vi "SampleAccumulator.vi"(7 "Write Element Data":T4={"Write Index"=0, "Write Element"=0, "Write?"=TRUE}, 8 "Input Valid":bool=TRUE, 9 "Acquisition Status In":T1, 11 "Input Data":T2=[0, 0, 0, 0]) -> (0 "End of Acc?":bool, 1 "Line Status Out":T3, 2 "Final Count":i16, 3 "Accumulated Value":i32[](array[numeric]), 5 "IsCurrentMaskNeg?":bool)   [LabVIEW 2014]
uses:
  <vilib>/rvi/FXPMathLib/basic elements/FxpDiscreteDelay/XNode/nifxpmath_DiscreteDelay.xnode
  <vilib>/rvi/DataTransferAndStorage/Container/XNode/niFpgaContainer.xnode
  <vilib>/rvi/interface/RandomDataEmulation/nirviRandomDataFpgaReadWriteTemplate.vi
  Adapter Module Specific/Multi-Channel Analog Input Data.ctl
  Acquisition Engine/Acquisition Status.ctl
panel:
  # "Copyright 2014 Vidrio Technologies\nScanImage 5 software is licensed under the Apache License, Version 2.0 (the \"License\"); you may not use any files contained\nwithin the ScanImage 5 release except in compliance with the License. You may obtain a copy of the License at\n http://www.apache.org/licenses/LICENSE-2.0\nUnless required by applicable law or agreed to in writing, software distributed under the License is distributed on an\n\"AS IS\" BASIS, WITHOUT WARRANTIES OR CONDITIONS OF ANY KIND, either express or implied. See the License for the\n specific language governing permissions and limitations under the License."
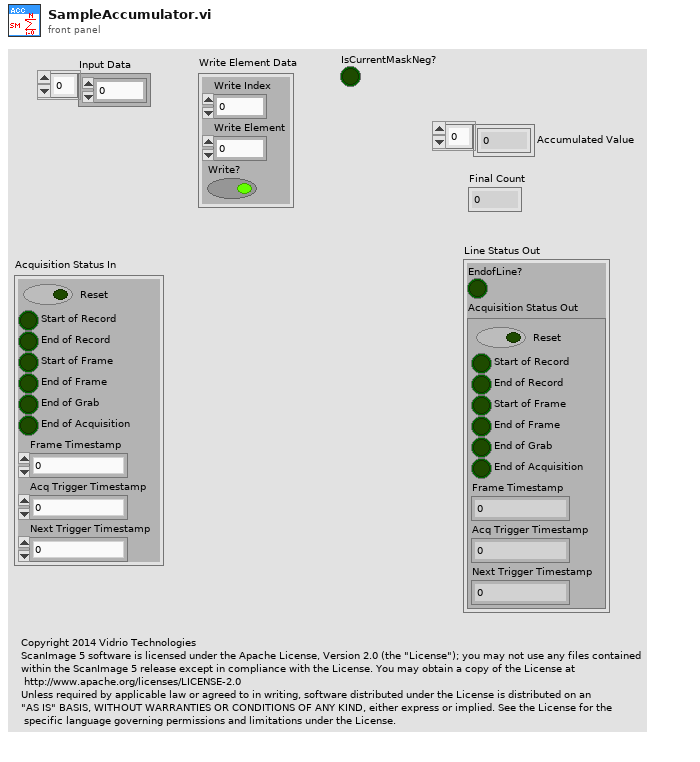
[diagram p1: front panel]
types:
  T1 = typedef "Acquisition Status.ctl" = cluster{"Reset":bool, "Start of Record":bool, "End of Record":bool, "Start of Frame":bool, "End of Frame":bool, "End of Grab":bool, "End of Acquisition":bool, "Frame Timestamp":u64, "Acq Trigger Timestamp":u64, "Next Trigger Timestamp":u64}
  T2 = typedef "Multi-Channel Analog Input Data.ctl" = i16[]
  T3 = cluster{"EndofLine?":bool, "Acquisition Status Out":T1}
  T4 = cluster{"Write Index":i32, "Write Element":i16, "Write?":bool}
  T5 = cluster{"Reset":bool, "Start of Record":bool, "End of Record":bool, "Start of Frame":bool, "End of Frame":bool, "End of Grab":bool, "End of Acquisition":bool, "Frame Timestamp":u64, "Acq Trigger Timestamp":u64, "Next Trigger Timestamp":u64}
  T6 = cluster{bool, "Q":cluster{"Reset":bool, "Start of Record":bool, "End of Record":bool, "Start of Frame":bool, "End of Frame":bool, "End of Grab":bool, "End of Acquisition":bool, "Frame Timestamp":u64, "Acq Trigger Timestamp":u64, "Next Trigger Timestamp":u64}}
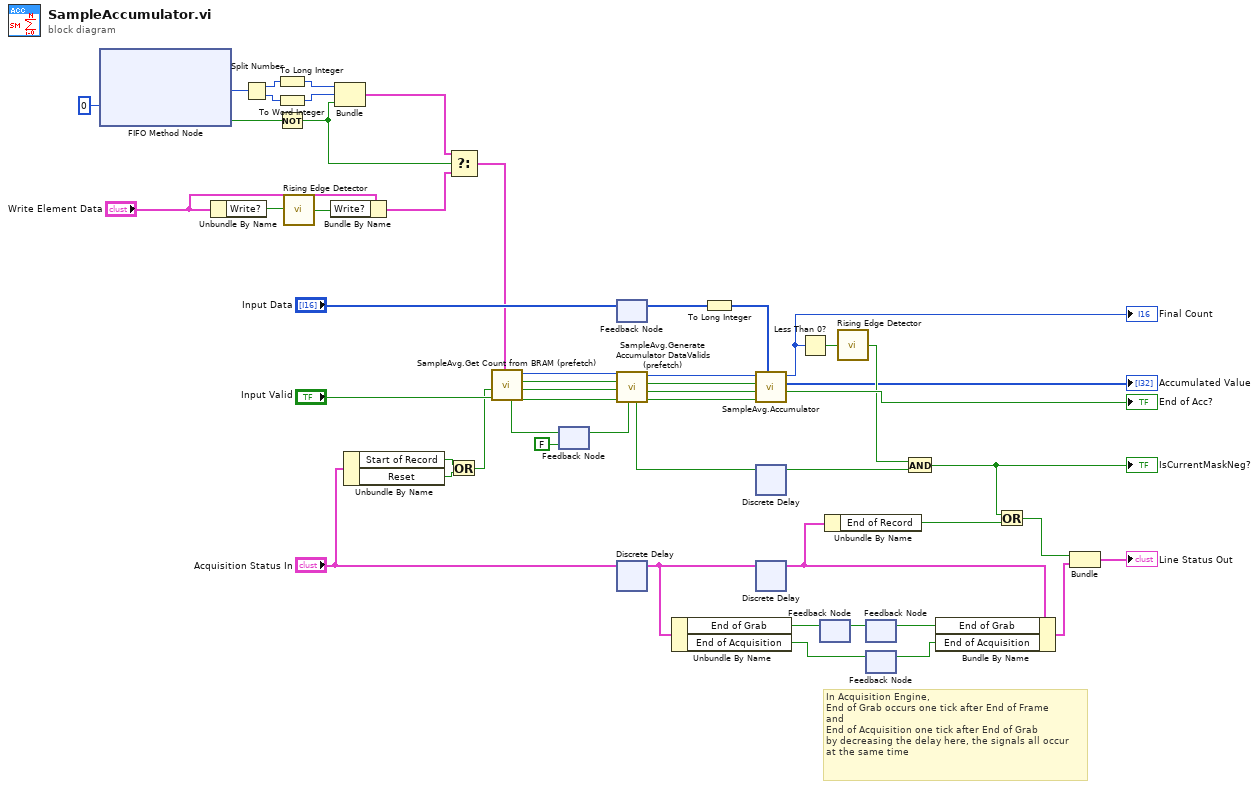
[diagram p0: block diagram]
diagram:
  # "In Acquisition Engine,\nEnd of Grab occurs one tick after End of Frame\nand\nEnd of Acquisition one tick after End of Grab\nby decreasing the delay here, the signals all occur\nat the same time"
  n1 = xnode ("FIFO Method Node")("Timeout"=0) -> ("Element"=w26:u32, "Timed Out?"=w23:bool)  [unwired: 1 in, 1 out]
  n2 = Unbundle By Name("Write Element Data") -> ("Write?"=w20:bool)
  n3 = Split Number(x=w26) -> (hi(x)=w22:u16, lo(x)=w25:u16)
  n4 = To Long Integer(number=w22) -> (32bit integer=w21:i32)
  n5 = To Word Integer(number=w25) -> (16bit integer=w24:i16)
  n6 = Not(x=w23) -> (.not. x?=w15:bool)
  n7 = call "Rising Edge Detector.vi"("signal"=w20) -> ("edge detected"=w18:bool)  [unwired: 14 in]
  n8 = Bundle By Name(cluster="Write Element Data", "Write?"=w18) -> (w17:T4)
  n9 = Bundle(w21, w24, w15) -> (w16:cluster{i32, i16, bool})  [unwired: 1 in]
  n10 = Unbundle By Name("Acquisition Status In") -> ("Start of Record"=w2:bool, "Reset"=w3:bool)
  n11 = Select(t=w16, s=w15, f=w17) -> (s? t:f=w14:T4)
  n12 = Or(x=w2, y=w3) -> (x .or. y?=w1:bool)
  n13 = feedback #1(FALSE ("Get New Load")) -> (w50:bool)
  n14 = call "SampleAvg.Get Count from BRAM (prefetch).vi"("Step?"=w50, "Write Element Data"=w14, "Input Valid"="Input Valid", "Start New Record"=w1) -> ("Output Valid"=w52:bool, "Start of New Record"=w47:bool, "NewCount?"=w48:bool, "Next Valid Counts"=w44:i16)  [unwired: 3 in, 1 out]
  n15 = feedback #2() -> (w29:T2)  [unwired: 1 in]
  n16 = feedback-in #2("Input Data") -> ()
  n17 = call "SampleAvg.Generate Accumulator DataValids (prefetch).vi"("Input Valid"=w52, "New Record?"=w47, "Load New Count"=w48, "Count"=w44) -> ("Output Valid"=w34:bool, "New Record"=w46:bool, "NewCount?"=w43:bool, "Count"=w42:i16, "WasInputValid?"=w33:bool, "Get New Load"=w45:bool)  [unwired: 2 in]
  n18 = feedback-in #1(w45) -> ()
  n19 = xnode "Discrete Delay"("D"="Acquisition Status In") -> ("Q"=w11:T5)
  n20 = Unbundle By Name(w11) -> ("End of Grab"=w10:bool, "End of Acquisition"=w8:bool)
  n21 = To Long Integer(number=w29) -> (32bit integer=w28:i32[])
  n22 = call "SampleAvg.Accumulator.vi"("Data"=w28, "Input Valid"=w34, "New Record"=w46, "NewCount?"=w43, "Count"=w42) -> ("Acc Valid"=→"End of Acc?":bool, "Accumulator"=→"Accumulated Value":i32[], "End Count"=w35:i16)  [unwired: 4 in]
  "Final Count" <- w35
  n23 = xnode "Discrete Delay"("D"=w33) -> ("Q"=w32:bool)
  n24 = xnode "Discrete Delay"("D"=w11) -> ("Q"=w7:T5)
  n25 = Less Than 0?(x=w35) -> (x < 0?=w40:bool)
  n26 = feedback-in #3(w10) -> ()
  n27 = feedback #3() -> (w9:bool)  [unwired: 1 in]
  n28 = Unbundle By Name(w7) -> ("End of Record"=w37:bool)
  n29 = call "Rising Edge Detector.vi"("signal"=w40) -> ("edge detected"=w39:bool)  [unwired: 14 in]
  n30 = feedback #4() -> (w5:bool)  [unwired: 1 in]
  n31 = feedback-in #4(w9) -> ()
  n32 = feedback #5() -> (w4:bool)  [unwired: 1 in]
  n33 = feedback-in #5(w8) -> ()
  n34 = And(x=w39, y=w32) -> (x .and. y?=w38:bool)
  "IsCurrentMaskNeg?" <- w38
  n35 = Bundle By Name(cluster=w7, "End of Grab"=w5, "End of Acquisition"=w4) -> (w6:T5)
  n36 = Or(x=w38, y=w37) -> (x .or. y?=w36:bool)
  n37 = Bundle(w36, "Q"=w6) -> (→"Line Status Out":T6)  [unwired: 1 in]
